vi "Average Angle (SubVI).vi"(1 "angles":dbl[](array[numeric])) -> (8 "average angle":dbl, 9 "fatal angle error?":bool, 10 "angle error?":bool)   [LabVIEW 2017]
doc: "Vi, na podstawie trzech wyliczyonych kątów, liczy wartość kąta dla środka urządzenia."
uses:
  Custom Controls/#typedef_AgleError_Enum.ctl
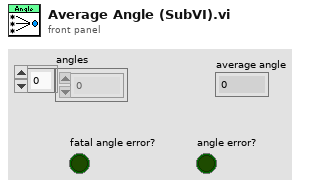
[diagram p1: front panel]
types:
  T1 = typedef "#typedef_AgleError_Enum.ctl" = enum16{"no error", "alpha error", "beta error", "gamma error", "fatal error"}
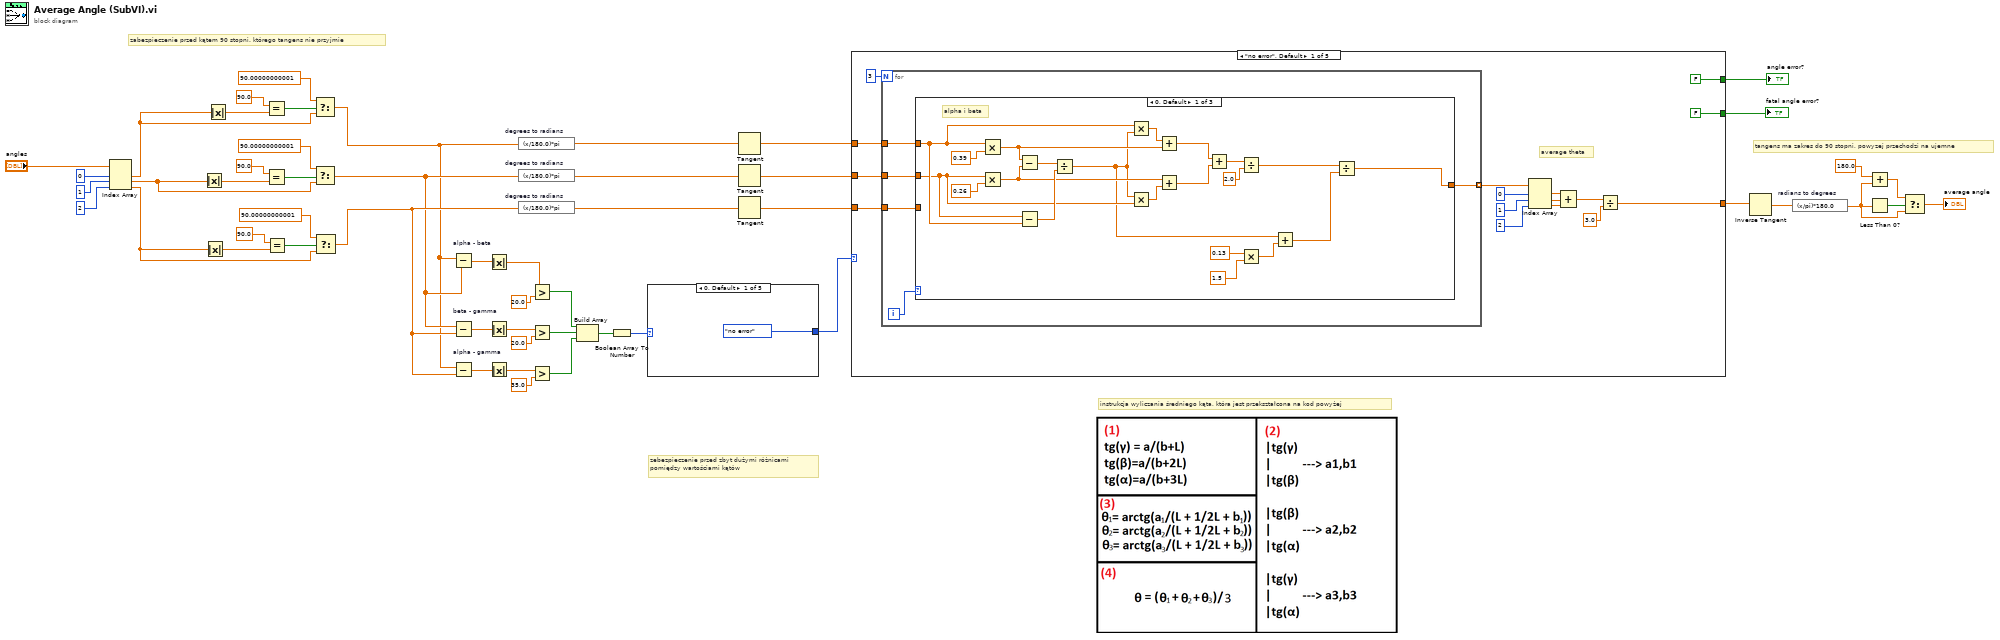
[diagram p0: block diagram]
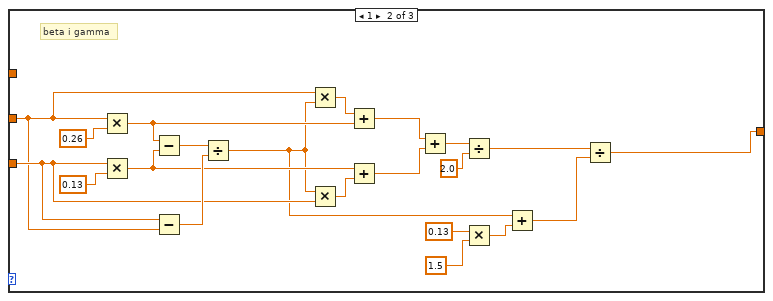
[diagram p2: hidden frame]
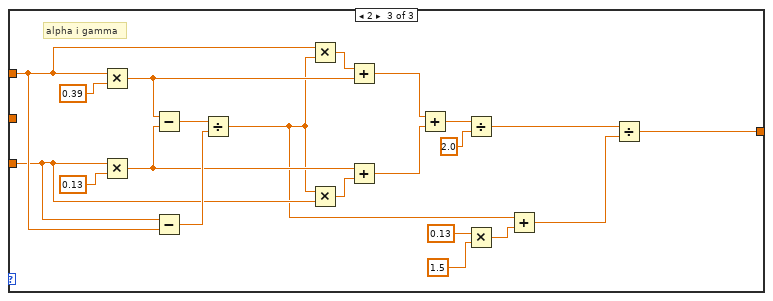
[diagram p3: hidden frame]
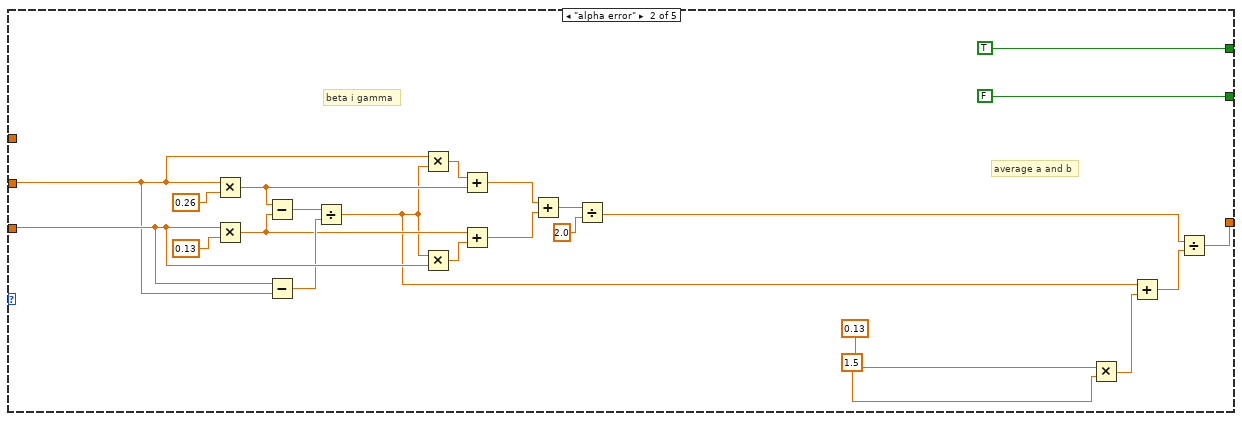
[diagram p4: hidden frame]
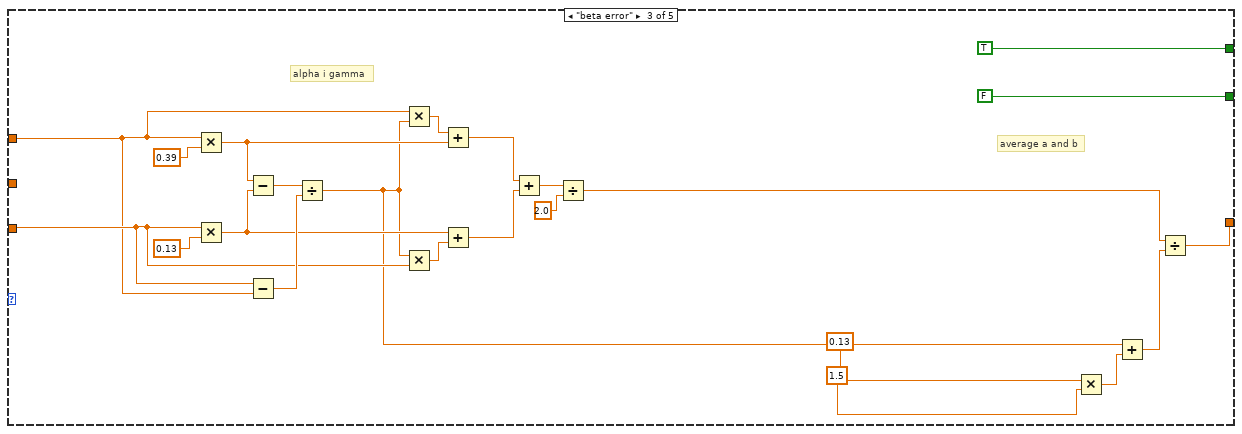
[diagram p5: hidden frame]
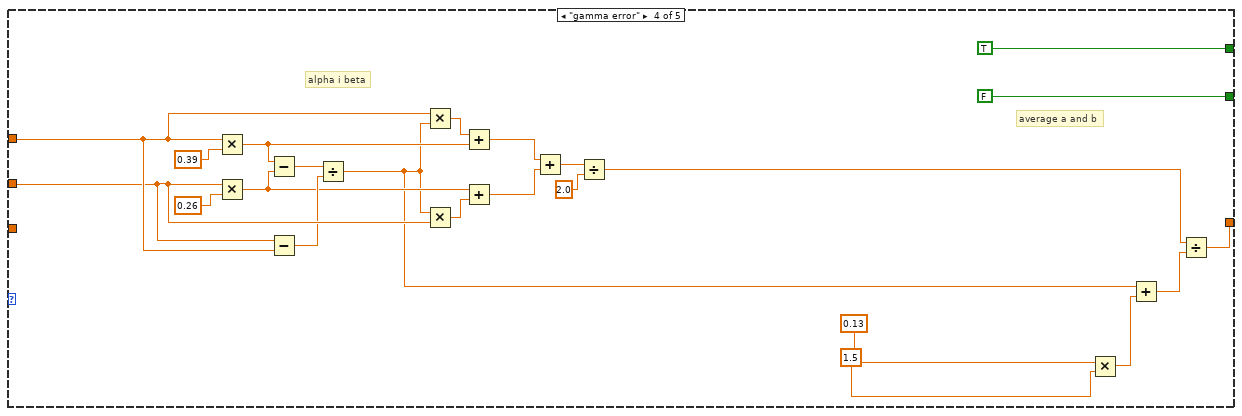
[diagram p6: hidden frame]
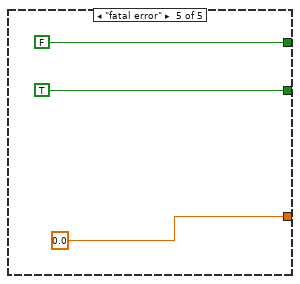
[diagram p7: hidden frame]
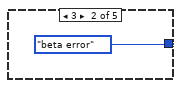
[diagram p8: hidden frame]
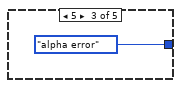
[diagram p9: hidden frame]
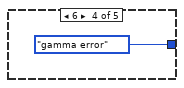
[diagram p10: hidden frame]
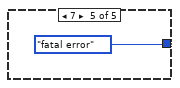
[diagram p11: hidden frame]
diagram:
  # "zabezpieczenie przed kątem 90 stopni. którego tangens nie przyjmie"
  # "zebezpieczenie przed zbyt dużymi różnicami \npomiędzy wartościami kątów"
  # "tangens ma zakres do 90 stopni, powyzej przechodzi na ujemne"
  # "instrukcja wyliczania średniego kąta, która jest przekształcona na kod powyżej"
  n1 = Index Array(array="angles", index #1=0 ("index"), index #2=1 ("index"), index #3=2 ("index")) -> (element #1=w8:dbl, element #2=w3:dbl, element #3=w11:dbl)
  n2 = Absolute Value(x=w3) -> (abs(x)=w7:dbl)
  n3 = Absolute Value(x=w11) -> (abs(x)=w10:dbl)
  n4 = Absolute Value(x=w8) -> (abs(x)=w16:dbl)
  n5 = Equal?(x=90.0 ("y"), y=w16) -> (x = y?=w19:bool)
  n6 = Equal?(x=90.0 ("y"), y=w7) -> (x = y?=w6:bool)
  n7 = Equal?(x=90.0 ("y"), y=w10) -> (x = y?=w13:bool)
  n8 = Select(t=90.00000000001, s=w19, f=w8) -> (s? t:f=w1:dbl)
  n9 = Select(t=90.00000000001, s=w6, f=w3) -> (s? t:f=w2:dbl)
  n10 = Select(t=90.00000000001, s=w13, f=w11) -> (s? t:f=w12:dbl)
  n11 = Subtract "alpha - beta"(x=w1, y=w2) -> (x-y=w39:dbl)
  n12 = Subtract "beta - gamma"(x=w2, y=w12) -> (x-y=w37:dbl)
  n13 = Subtract "alpha - gamma"(x=w1, y=w12) -> (x-y=w38:dbl)
  n14 = Absolute Value(x=w39) -> (abs(x)=w36:dbl)
  n15 = Absolute Value(x=w37) -> (abs(x)=w33:dbl)
  n16 = Absolute Value(x=w38) -> (abs(x)=w31:dbl)
  n17 = expression code="(x/180.0)*pi" "degrees to radians"(w1) -> (w25:dbl)
  n18 = expression code="(x/180.0)*pi" "degrees to radians"(w2) -> (w24:dbl)
  n19 = expression code="(x/180.0)*pi" "degrees to radians"(w12) -> (w23:dbl)
  n20 = Greater?(x=w36, y=20.0) -> (0:w28:bool)
  n21 = Greater?(x=w33, y=20.0) -> (0:w30:bool)
  n22 = Greater?(x=w31, y=35.0) -> (0:w29:bool)
  n23 = Build Array(w28, w30, w29) -> (w27:bool[])
  n24 = Boolean Array To Number(Boolean array=w27) -> (number=w26:u32)
  n25 = case shown="0, Default" w26 {
    tunnel: [#typedef_AgleError_Enum."no error" ("Enum") #typedef_AgleError_Enum."beta error" ("Enum") #typedef_AgleError_Enum."alpha error" ("Enum") #typedef_AgleError_Enum."gamma error" ("Enum") #typedef_AgleError_Enum."fatal error" ("Enum")] -> w22
    frame 0, Default {
    }
    frame 3 {
    }
    frame 5 {
    }
    frame 6 {
    }
    frame 7 {
    }
  }
  n26 = Tangent(1:w25) -> (0:w50:dbl)
  n27 = Tangent(1:w24) -> (0:w51:dbl)
  n28 = Tangent(1:w23) -> (0:w52:dbl)
  n29 = case shown="\"no error\", Default" w22 {
    tunnel: w52 -> [w73 w159 w170 _ _]
    tunnel: w51 -> [w72 w158 _ w204 _]
    tunnel: w50 -> [w71 _ w169 w205 _]
    tunnel: [w58 w160 w183 w206 0.0] -> w45
    tunnel: [FALSE FALSE FALSE FALSE TRUE] -> w21
    tunnel: [FALSE TRUE TRUE TRUE FALSE] -> w20
    frame "no error", Default {
      # "average theta"
      n30 = for {
        N: 3 -> [_]
        tunnel: w71 -> [w77]
        tunnel: w72 -> [w76]
        tunnel: w73 -> [w75]
        tunnel: [w74] -> w65 mode=indexing
        i -> [w78]
        n31 = case shown="0, Default" w78 {
          tunnel: w77 -> [w95 _ w137]
          tunnel: w76 -> [w91 w107 _]
          tunnel: w75 -> [_ w108 w128]
          tunnel: [w79 w100 w121] -> w74
          frame 0, Default {
            # "alpha i beta"
            n32 = Multiply(x=w95, y=0.39) -> (x*y=w93:dbl)
            n33 = Multiply(x=w91, y=0.26) -> (x*y=w90:dbl)
            n34 = Subtract(x=w93, y=w90) -> (x-y=w97:dbl)
            n35 = Subtract(x=w91, y=w95) -> (x-y=w96:dbl)
            n36 = Divide(x=w97, y=w96) -> (x/y=w80:dbl)
            n37 = Multiply(x=w95, y=w80) -> (x*y=w94:dbl)
            n38 = Multiply(x=w80, y=w91) -> (x*y=w92:dbl)
            n39 = Add(x=w94, y=w93) -> (x+y=w89:dbl)
            n40 = Add(x=w90, y=w92) -> (x+y=w88:dbl)
            n41 = Add(x=w89, y=w88) -> (x+y=w87:dbl)
            n42 = Divide(x=w87, y=2.0) -> (x/y=w82:dbl)
            n43 = Multiply(x=0.13, y=1.5) -> (x*y=w84:dbl)
            n44 = Add(x=w80, y=w84) -> (x+y=w83:dbl)
            n45 = Divide(x=w82, y=w83) -> (x/y=w79:dbl)
          }
          frame 1 {
            # "beta i gamma"
            n46 = Multiply(x=w107, y=0.26) -> (x*y=w115:dbl)
            n47 = Multiply(x=w108, y=0.13) -> (x*y=w113:dbl)
            n48 = Subtract(x=w115, y=w113) -> (x-y=w118:dbl)
            n49 = Subtract(x=w108, y=w107) -> (x-y=w117:dbl)
            n50 = Divide(x=w118, y=w117) -> (x/y=w102:dbl)
            n51 = Multiply(x=w107, y=w102) -> (x*y=w116:dbl)
            n52 = Multiply(x=w102, y=w108) -> (x*y=w114:dbl)
            n53 = Add(x=w116, y=w115) -> (x+y=w112:dbl)
            n54 = Add(x=w113, y=w114) -> (x+y=w111:dbl)
            n55 = Add(x=w112, y=w111) -> (x+y=w110:dbl)
            n56 = Divide(x=w110, y=2.0) -> (x/y=w106:dbl)
            n57 = Multiply(x=0.13, y=1.5) -> (x*y=w103:dbl)
            n58 = Add(x=w102, y=w103) -> (x+y=w101:dbl)
            n59 = Divide(x=w106, y=w101) -> (x/y=w100:dbl)
          }
          frame 2 {
            # "alpha i gamma"
            n60 = Multiply(x=w137, y=0.39) -> (x*y=w135:dbl)
            n61 = Multiply(x=w128, y=0.13) -> (x*y=w133:dbl)
            n62 = Subtract(x=w135, y=w133) -> (x-y=w139:dbl)
            n63 = Subtract(x=w128, y=w137) -> (x-y=w138:dbl)
            n64 = Divide(x=w139, y=w138) -> (x/y=w122:dbl)
            n65 = Multiply(x=w137, y=w122) -> (x*y=w136:dbl)
            n66 = Multiply(x=w122, y=w128) -> (x*y=w134:dbl)
            n67 = Add(x=w136, y=w135) -> (x+y=w132:dbl)
            n68 = Add(x=w133, y=w134) -> (x+y=w131:dbl)
            n69 = Add(x=w132, y=w131) -> (x+y=w130:dbl)
            n70 = Divide(x=w130, y=2.0) -> (x/y=w124:dbl)
            n71 = Multiply(x=0.13, y=1.5) -> (x*y=w126:dbl)
            n72 = Add(x=w122, y=w126) -> (x+y=w125:dbl)
            n73 = Divide(x=w124, y=w125) -> (x/y=w121:dbl)
          }
        }
      }
      n74 = Index Array(array=w65, index #1=0 ("index"), index #2=1 ("index"), index #3=2 ("index")) -> (element #1=w68:dbl, element #2=w66:dbl, element #3=w67:dbl)
      n75 = Compound Arithmetic op=ADD(w68, w66, w67) -> (w69:dbl)
      n76 = Divide(x=w69, y=3.0) -> (x/y=w58:dbl)
    }
    frame "alpha error" {
      # "beta i gamma"
      # "average a and b"
      n77 = Multiply(x=w158, y=0.26) -> (x*y=w152:dbl)
      n78 = Multiply(x=w159, y=0.13) -> (x*y=w150:dbl)
      n79 = Subtract(x=w152, y=w150) -> (x-y=w155:dbl)
      n80 = Subtract(x=w159, y=w158) -> (x-y=w154:dbl)
      n81 = Divide(x=w155, y=w154) -> (x/y=w144:dbl)
      n82 = Multiply(x=w158, y=w144) -> (x*y=w153:dbl)
      n83 = Multiply(x=w144, y=w159) -> (x*y=w151:dbl)
      n84 = Add(x=w153, y=w152) -> (x+y=w149:dbl)
      n85 = Add(x=w150, y=w151) -> (x+y=w148:dbl)
      n86 = Add(x=w149, y=w148) -> (x+y=w147:dbl)
      n87 = Divide(x=w147, y=2.0) -> (x/y=w145:dbl)
      n88 = Multiply(x=0.13, y=1.5) -> (x*y=w164:dbl)
      n89 = Add(x=w144, y=w164) -> (x+y=w161:dbl)
      n90 = Divide(x=w145, y=w161) -> (x/y=w160:dbl)
    }
    frame "beta error" {
      # "alpha i gamma"
      # "average a and b"
      n91 = Multiply(x=w169, y=0.39) -> (x*y=w177:dbl)
      n92 = Multiply(x=w170, y=0.13) -> (x*y=w175:dbl)
      n93 = Subtract(x=w177, y=w175) -> (x-y=w180:dbl)
      n94 = Subtract(x=w170, y=w169) -> (x-y=w179:dbl)
      n95 = Divide(x=w180, y=w179) -> (x/y=w168:dbl)
      n96 = Multiply(x=w169, y=w168) -> (x*y=w178:dbl)
      n97 = Multiply(x=w168, y=w170) -> (x*y=w176:dbl)
      n98 = Add(x=w178, y=w177) -> (x+y=w174:dbl)
      n99 = Add(x=w175, y=w176) -> (x+y=w173:dbl)
      n100 = Add(x=w174, y=w173) -> (x+y=w172:dbl)
      n101 = Divide(x=w172, y=2.0) -> (x/y=w167:dbl)
      n102 = Multiply(x=0.13, y=1.5) -> (x*y=w187:dbl)
      n103 = Add(x=w168, y=w187) -> (x+y=w184:dbl)
      n104 = Divide(x=w167, y=w184) -> (x/y=w183:dbl)
    }
    frame "gamma error" {
      # "alpha i beta"
      # "average a and b"
      n105 = Multiply(x=w205, y=0.39) -> (x*y=w198:dbl)
      n106 = Multiply(x=w204, y=0.26) -> (x*y=w196:dbl)
      n107 = Subtract(x=w198, y=w196) -> (x-y=w201:dbl)
      n108 = Subtract(x=w204, y=w205) -> (x-y=w200:dbl)
      n109 = Divide(x=w201, y=w200) -> (x/y=w191:dbl)
      n110 = Multiply(x=w205, y=w191) -> (x*y=w199:dbl)
      n111 = Multiply(x=w191, y=w204) -> (x*y=w197:dbl)
      n112 = Add(x=w199, y=w198) -> (x+y=w195:dbl)
      n113 = Add(x=w196, y=w197) -> (x+y=w194:dbl)
      n114 = Add(x=w195, y=w194) -> (x+y=w193:dbl)
      n115 = Divide(x=w193, y=2.0) -> (x/y=w190:dbl)
      n116 = Multiply(x=0.13, y=1.5) -> (x*y=w210:dbl)
      n117 = Add(x=w191, y=w210) -> (x+y=w207:dbl)
      n118 = Divide(x=w190, y=w207) -> (x/y=w206:dbl)
    }
    frame "fatal error" {
    }
  }
  "fatal angle error?" <- w21
  "angle error?" <- w20
  n119 = Inverse Tangent(1:w45) -> (0:w46:dbl)
  n120 = expression code="(x/pi)*180.0" "radians to degrees"(w46) -> (w42:dbl)
  n121 = Add(x=180.0, y=w42) -> (x+y=w41:dbl)
  n122 = Less Than 0?(x=w42) -> (x < 0?=w44:bool)
  n123 = Select(t=w41, s=w44, f=w42) -> (s? t:f=→"average angle":dbl)
